vi "Terminate.vi"(11 "Terminate":T1=enum."ReInit") -> ()   [LabVIEW 2013, in "ToplevelControllerLibrary.lvlib"]
uses:
  ToplevelControllerLibrary.lvlib
  Private Controls/Terminate.ctl
  Modules/UserConsole/PrivateControls/UserConsole_QueueDriver.ctl
  Modules/DisplayConsole/PrivateContols/DisplayConsole_QueueDriver.ctl
  Modules/SensorConsole/PrivateControls/SensorConsole_QueueDriver.ctl
  Modules/UserConsole/UserConsole.lvlib
  Modules/DisplayConsole/DisplayConsoleLib.lvlib
  Modules/SensorConsole/SensorConsoleLib.lvlib
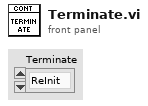
[diagram p1: front panel]
types:
  T1 = typedef "ToplevelControllerLibrary.lvlib/Terminate.ctl" = enum16{"Update UserConsole", "Update DisplayConsole", "ReInit"}
  T2 = typedef "UserConsole.lvlib/UserConsole_QueueDriver.ctl" = enum16{"Default Case", "Init", "Enqueue", "Dequeue", "ReleaseQueue", "Exit"}
  T3 = typedef "DisplayConsoleLib.lvlib/DisplayConsole_QueueDriver.ctl" = enum16{"Default Case", "Init", "Enqueue", "Dequeue", "ReleaseQueue", "Exit"}
  T4 = enum16{"Init", "Enqueue", "Dequeue", "ReleaseQueue", "Exit"}
  T5 = typedef "SensorConsoleLib.lvlib/SensorConsole_QueueDriver.ctl" = enum16{"Default case", "Init", "Enqueue", "Dequeue", "ReleaseQueue", "Exit"}
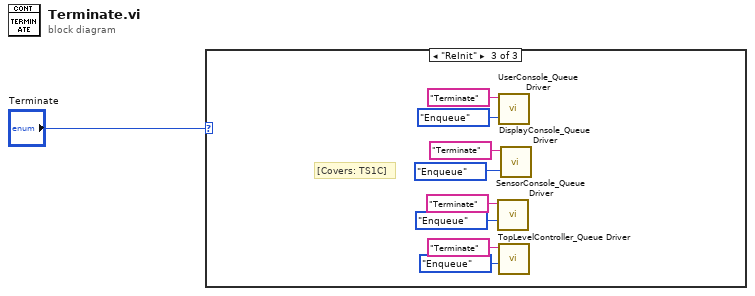
[diagram p0: block diagram]
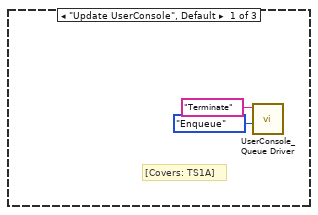
[diagram p2: hidden frame]
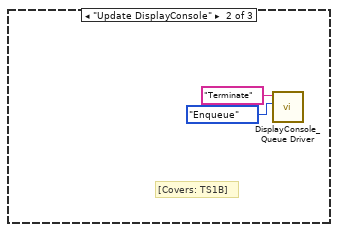
[diagram p3: hidden frame]
diagram:
  n1 = case shown="\"ReInit\"" "Terminate" {
    frame "Update UserConsole", Default {
      # "[Covers: TS1A]"
      n2 = call "UserConsole_Queue Driver.vi"("State"=UserConsole_QueueDriver."Enqueue", "EnQ"="Terminate") -> ()  [unwired: 8 in, 2 out]
    }
    frame "Update DisplayConsole" {
      # "[Covers: TS1B]"
      n3 = call "DisplayConsole_Queue Driver.vi"("State"=DisplayConsole_QueueDriver."Enqueue", "EnQ"="Terminate") -> ()  [unwired: 8 in, 2 out]
    }
    frame "ReInit" {
      # "[Covers: TS1C]"
      n4 = call "SensorConsole_Queue Driver.vi"("Enum"=SensorConsole_QueueDriver."Enqueue", "EnQ"="Terminate") -> ()  [unwired: 8 in, 2 out]
      n5 = call "UserConsole_Queue Driver.vi"("State"=UserConsole_QueueDriver."Enqueue", "EnQ"="Terminate") -> ()  [unwired: 8 in, 2 out]
      n6 = call "TopLevelController_Queue Driver.vi"("Enum"=T4."Enqueue", "EnQ"="Terminate") -> ()  [unwired: 8 in, 2 out]
      n7 = call "DisplayConsole_Queue Driver.vi"("State"=DisplayConsole_QueueDriver."Enqueue", "EnQ"="Terminate") -> ()  [unwired: 8 in, 2 out]
    }
  }
